vi "PH_uOPA_DelayController.constructor.vi"(0 "name":string, 2 "data in":string, 5 "error in(no error)":errorcluster) -> (14 "i ref out":refnum<vi>, 16 "data out":string, 19 "error out":errorcluster)   [LabVIEW 2014, in "PH_uOPA_DelayController.lvlib"]
doc: "This is the constructor of a class.\n\nLicense Agreement for this software:\n\nCopyright (C)\nGesellschaft für Schwerionenforschung, GSI\nPlanckstr. 1\n64291 Darmstadt\nGermany\n\nContact: D.Beck@gsi.de \n\nThis program is free software; you can redistribute it and/or modify it under the terms of the \nGNU General Public License as published by the Free Software Foundation; either version 2 of \nthe license, or (at your option) any later version.\n\nThis program is distributed in the hope that it will be useful, but WITHOUT ANY WARRANTY; \nwithout even the implied warranty of MERCHANTABILITY or FITNESS FOR A PARTICULAR PURPOSE. See the GNU General License for more details (http://www.gnu.org).\n\nGesellschaft für Schwerionenforschung, GSI\nPlanckstr. 1, 64291 Darmstadt, Germany\nFor all questions and ideas contact: M.Richter@gsi.de, H.Brand@gsi.de or D.Beck@gsi.de.\nLast update: 16-JUN-2004"
uses:
  PH_uOPA_DelayController.lvlib
  CS_Core/CSSystem/CSSystemLib/CSSystemLib.lvlib
  PH_Devices/PH_TKTDS-30xx/PH_TKTDS-30xx.lvlib
  CS_Core/CSObj/CSObj.lvlib
  PH_Basics/PH_Class/PH_Class.lvlib
  PH_Basics/PH_StatusHandler/PH_StatusHandler.lvlib
  PH_Basics/PH_AxisGUI_BaseClass/PH_AxisGUI_BaseClass.lvlib
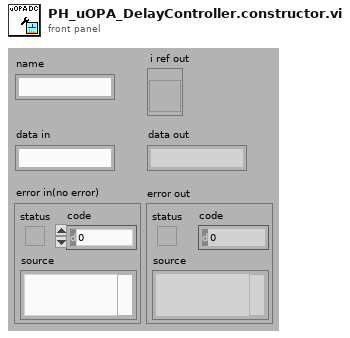
[diagram p1: front panel]
types:
  T1 = enum16{"SetAttribute", "GetAttribute", "CreateAttribute", "DestroyAttribute", "DestroyAllAtributes"}
  T2 = typedef "PH_uOPA_DelayController.lvlib/PH_uOPA_DelayController.i attribute.ctl" = cluster{"GUI Refs":cluster{"Current Pump Peak":refnum<vi>, "Current uOPA Peak":refnum<vi>, "Pump Peak":refnum<vi>, "uOPA Peak":refnum<vi>, "uOPA Target":refnum<vi>, "uOPA Limits [%]":refnum<vi>, "sample length":refnum<vi>, "Pump Target":refnum<vi>, "Pump Limit":refnum<vi>, "Pump running":refnum<vi>, "Feedback Control":refnum<vi>, "Control Status":refnum<vi>, "uOPA Mean":refnum<vi>, "Current uOPA Mean":refnum<vi>}, "uOPA Target":dbl, "uOPA Limits [%]":T3, "Sample Length":i32, "Initialize Mean":bool, "Pump Target":dbl, "Pump Limit [%]":dbl, "Feedback Control":bool, "Control Status":T4, "last Mean":dbl, "last direction":T5, "Axis Settings":T6, "Width while feedback":dbl}
  T3 = typedef "PH_uOPA_DelayController.lvlib/PH_uOPA_DelayController.Limit.ctl" = cluster{"low":dbl, "activate":dbl, "fine":dbl}
  T4 = typedef "PH_uOPA_DelayController.lvlib/PH_uOPA_DelayController.Control Status.ctl" = enum32{"off", "Pump off", "calculating", "too low", "activated", "fine"}
  T5 = typedef "PH_Stepmotor_BaseClass.lvlib/PH_Stepmotor_BaseClass.Axis Direction.ctl" = enum16{"forward", "backward"}
  T6 = typedef "PH_Stepmotor_BaseClass.lvlib/PH_Stepmotor_BaseClass.Axis Settings.ctl" = cluster{"Sign change":bool, "Width":dbl, "Calibration":dbl, "Unit":string, "Motor Type":T7, "Unit Width":string, "Unit CF":string}
  T7 = typedef "PH_Stepmotor_BaseClass.lvlib/PH_Stepmotor_BaseClass.Motor Type.ctl" = enum16{"Unspecific", "OWIS 49.120.2633", "OWIS 49.060.1033", "OWIS 43.040.2558", "Diamond Motion 2200 series", "OWIS 49.120.266B.MV6", "Calorimeter", "Linear Stage 1", "MICOS VT-80", "MICOS VT-80 S", "Standa Rotstage nt0.95A", "PUF RA 320.200", "PUF RA 800.200", "PUF RA 800.400", "PUF RA 400.50", "1324.nn.800.50", "1324.n9c.800.50", "1324.nn.320.200", "1324.nn.400.200", "1324.nn.800.200", "1324.nn.400.50", "1324.8c9c.800.50", "1324.8c9c.400.200"}
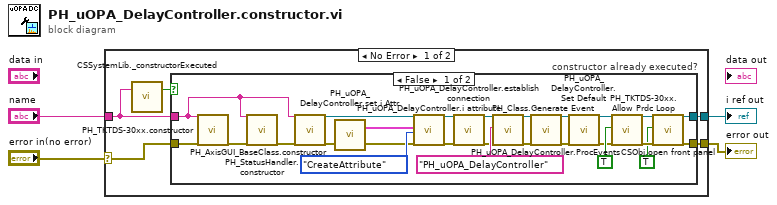
[diagram p0: block diagram]
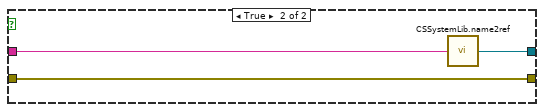
[diagram p2: hidden frame]
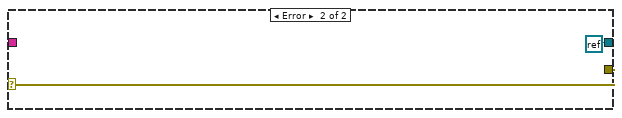
[diagram p3: hidden frame]
diagram:
  n1 = case shown="No Error" "error in(no error)" {
    selector: "error in(no error)" -> [w7 w39]
    tunnel: "name" -> [w6 _]
    tunnel: [w9 refnum<k0> refnum] -> w3
    tunnel: [w8 w39] -> w2
    frame No Error {
      n2 = call "CSSystemLib._constructorExecuted.vi"("name"=w6) -> ("constructor executed?"=w5:bool)  [unwired: 18 in]
      n3 = case "constructor already executed?" shown="False" w5 {
        tunnel: [w32 w37] -> w9
        tunnel: [w30 w36] -> w8
        tunnel: w7 -> [w15 w36]
        tunnel: w6 -> [w13 w38]
        frame False {
          n4 = call "PH_TKTDS-30xx.constructor.vi"("name"=w13, "error in(no error)"=w15) -> ("error out"=w25:errorcluster)  [unwired: 15 in, 2 out]
          n5 = call "PH_StatusHandler.constructor.vi"("name"=w13, "error in(no error)"=w25) -> ("error out"=w26:errorcluster)  [unwired: 15 in, 2 out]
          n6 = call "PH_AxisGUI_BaseClass.constructor.vi"("name"=w13, "error in(no error)"=w26) -> ("i ref out"=w14:refnum<vi>, "error out"=w12:errorcluster)  [unwired: 15 in, 1 out]
          n7 = call "PH_uOPA_DelayController.set i Attr.vi"("error in(no error)"=w12) -> ("error out"=w11:errorcluster, "i Attr"=w10:T2)  [unwired: 1 in]
          n8 = call "PH_uOPA_DelayController.i attribute.vi"("VI Refnum"=w14, "CLASS.i attribute"=w10, "Action"=T1."CreateAttribute", "error in (no error)"=w11) -> ("VI Refnum out"=w24:refnum<vi>, "error out"=w23:errorcluster)  [unwired: 13 in, 1 out]
          n9 = call "PH_uOPA_DelayController.establish connection.vi"("i ref in"=w24, "error in"=w23) -> ("i ref out"=w17:refnum<vi>, "error out"=w16:errorcluster)  [unwired: 16 in]
          n10 = call "PH_Class.Generate Event.vi"("i ref in"=w17, "Class"="PH_uOPA_DelayController", "error in (no error)"=w16) -> ("i ref out"=w22:refnum<vi>, "error out"=w21:errorcluster)  [unwired: 15 in]
          n11 = call "PH_uOPA_DelayController.ProcEvents.vi"("i ref in"=w22, "error in"=w21) -> ("i ref out"=w33:refnum<vi>, "error out"=w34:errorcluster)  [unwired: 16 in]
          n12 = call "PH_uOPA_DelayController.Set Default.vi"("i ref in"=w33, "error in"=w34) -> ("i ref out"=w19:refnum<vi>, "error out"=w18:errorcluster)  [unwired: 16 in]
          n13 = call "PH_TKTDS-30xx.Allow Prdc Loop.vi"("i ref in"=w19, "Allow Prdc Loop?"=TRUE ("Contructor finished"), "error in"=w18) -> ("i ref out"=w31:refnum<vi>, "error out"=w29:errorcluster)  [unwired: 15 in]
          n14 = call "CSObj.open front panel.vi"("i ref in"=w31, "frontPanelOpen"=TRUE, "error in (no error)"=w29) -> ("i ref out"=w32:refnum<vi>, "error out"=w30:errorcluster)  [unwired: 15 in]
        }
        frame True {
          n15 = call "CSSystemLib.name2ref.vi"("name"=w38) -> ("obj refnum"=w37:refnum<vi>)
        }
      }
    }
    frame Error {
    }
  }
  "i ref out" <- w3
  "error out" <- w2
